vi "SAOMM-BuildTypeArray.vi"(7 "command.ini":path) -> (8 "CommandArray":cluster{string[], u32[]})   [LabVIEW 2019]
uses:
  <vilib>/Utility/config.llb/Read Key (U32).vi
  <vilib>/Utility/config.llb/NI_LVConfig.lvlib
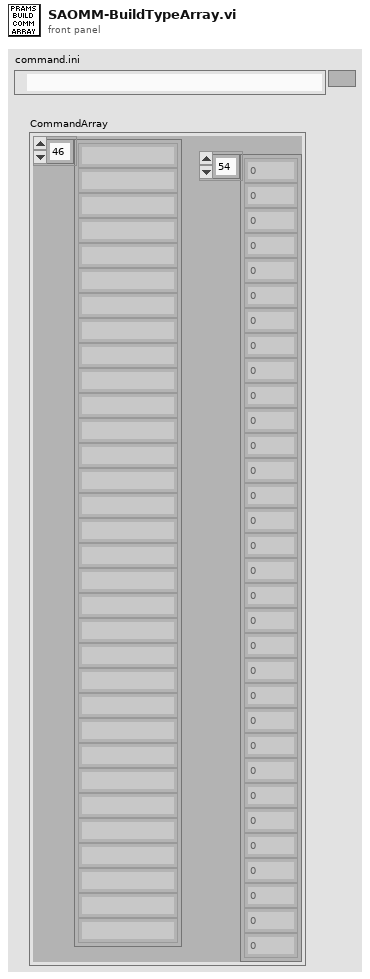
[diagram p1: front panel]
types:
  T1 = typedef "NI_LVConfig.lvlib/Config Data RefNum.ctl" = refnum<k1>
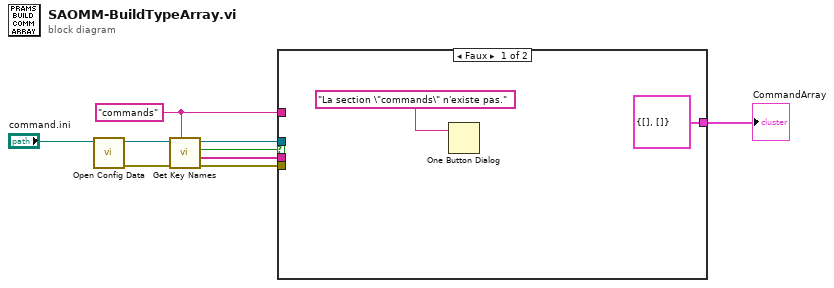
[diagram p0: block diagram]
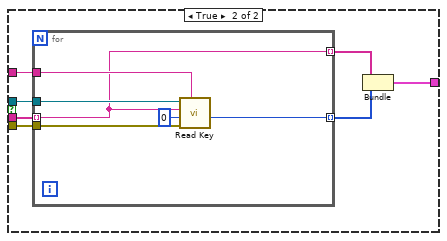
[diagram p2: hidden frame]
diagram:
  w4 = "commands" ("section")
  n1 = call <vilib>:"Open Config Data.vi"("configuration file path"="command.ini") -> ("error out"=w7:errorcluster, "refnum"=w8:T1)  [unwired: 8 in, 1 out]
  n2 = call <vilib>:"Get Key Names.vi"("section"=w4, "error in (no error)"=w7, "refnum"=w8) -> ("error out"=w2:errorcluster, "key names"=w5:string[], "section exists?"=w6:bool, "refnum out"=w3:T1)  [unwired: 5 in]
  n3 = case shown="Faux" w6 {
    tunnel: w5 -> [_ w16]
    tunnel: w4 -> [_ w18]
    tunnel: w3 -> [_ w17]
    tunnel: w2 -> [_ w15]
    tunnel: [cluster{string[], u32[]} {[], []} w12] -> w1
    frame False {
      n4 = One Button Dialog(message="La section \"commands\" n'existe pas.") -> ()  [unwired: 1 in, 1 out]
    }
    frame True {
      n5 = for {
        tunnel: w18 -> [w24]
        tunnel: w17 -> [w23]
        tunnel: w16 -> [w20] mode=indexing
        tunnel: w15 -> [w21]
        tunnel: [w20] -> w14 mode=indexing
        tunnel: [w19] -> w13 mode=indexing
        n6 = call-poly <vilib>:"Read Key.vi"("section"=w24, "error in (no error)"=w21, "default value"=u32 0, "key"=w20, "refnum"=w23) -> ("value"=w19:u32)  [unwired: 3 in, 3 out]
      }
      n7 = Bundle(w14, w13) -> (w12:cluster{string[], u32[]})  [unwired: 1 in]
    }
  }
  "CommandArray" <- w1
